vi "Test Panel.vi"() -> ()   [LabVIEW 2016]
uses:
  typedefs/Controlword--enum.ctl
  typedefs/Controlword--cluster.ctl
  typedefs/Statusword--cluster.ctl
  typedefs/Statusword--enum.ctl
  Libraries/Modbus-Master/MB_PDU/MB_PDU_Cluster.ctl
  IgusMotorDrive.lvclass
  Libraries/Modbus-Master/MB Master.lvlib
panel:
  out "Command":T1={"Function Code"=1, "Data"=[], "RTU_DataBytes"=0} {"Data" format="%.0x"}
  out "Response":T1={"Function Code"=1, "Data"=[], "RTU_DataBytes"=0} {"Data" format="%.0x"}
  in  "Stop Button":bool
  in  "Tab Control":T2(tab)
  in  "IP address":string="10.130.56.165"
  in  "port (502)":u16=502
  in  "Receive":bool
  in  "Send":bool
  in  "Controlword":T3=enum."Fault Reset"
  out "Controlword Out":T4
  out "Statusword out":T5
  out "Status":T6
  in  "Refresh Home Status":bool
  out "Homed Success":bool
  out "Homed":bool
  in  "Home":bool
  out "Actual Position":i32
  in  "Refresh Move Status":bool
  out "New Setpoint":bool
  in  "Move":bool
  in  "Setpoint Deceleration":u32
  in  "Setpoint Acceleration":u32=10000
  in  "Setpoint Velocity":u32=10000
  in  "Setpoint Position":i32=1000
  out "Target Reached":bool
  # "|    |    |    |    |    |    |    |    |    |    |    |    |    |    |\n|    |    |    |    |    |    |    |    |    |    |    +----+----+----+- Byte 19 ... 22: data field\n|    |    |    |    |    |    |    |    |    +----+- Byte 17, 18: SDO object bytes, = 1 ... 4\n|    |    |    |    |    |    |    +----+- Byte 15, 16: starting address = 0\n|    |    |    |    |    |    + Byte 14: sub index\n|    |    |    |    +----+- Byte 12, 13: object index\n|    |    |    +- Byte 11: Node ID = 0\n|    |    +------ Byte 10: protocol option fields, reserve, = 0\n|    +------ Byte  9: protocol option fields, 0 = read, 1 = write\n+----------- Byte  8 : MEI type, Modbus TCP = 13 (0Dh)"
  # "Set IP Address Run VI, if no error in connection, goto Initialisation"
  # "Status is polled continuously.\n\n\"Not ready to switch on\" and \"Switch On Disabled\" tell you that you should RTM and set Drive Profile to Modbus TCP before you set DI7/Enable.\n\nDepending upon Status select a suitable Controlword based on the transitions in the table below.\n\nOnce you have reached Operation Enabled, you may proceed to the Homing Mode tab."
  # "Click Home, stage should start homing\n\nClick Refresh to check status"
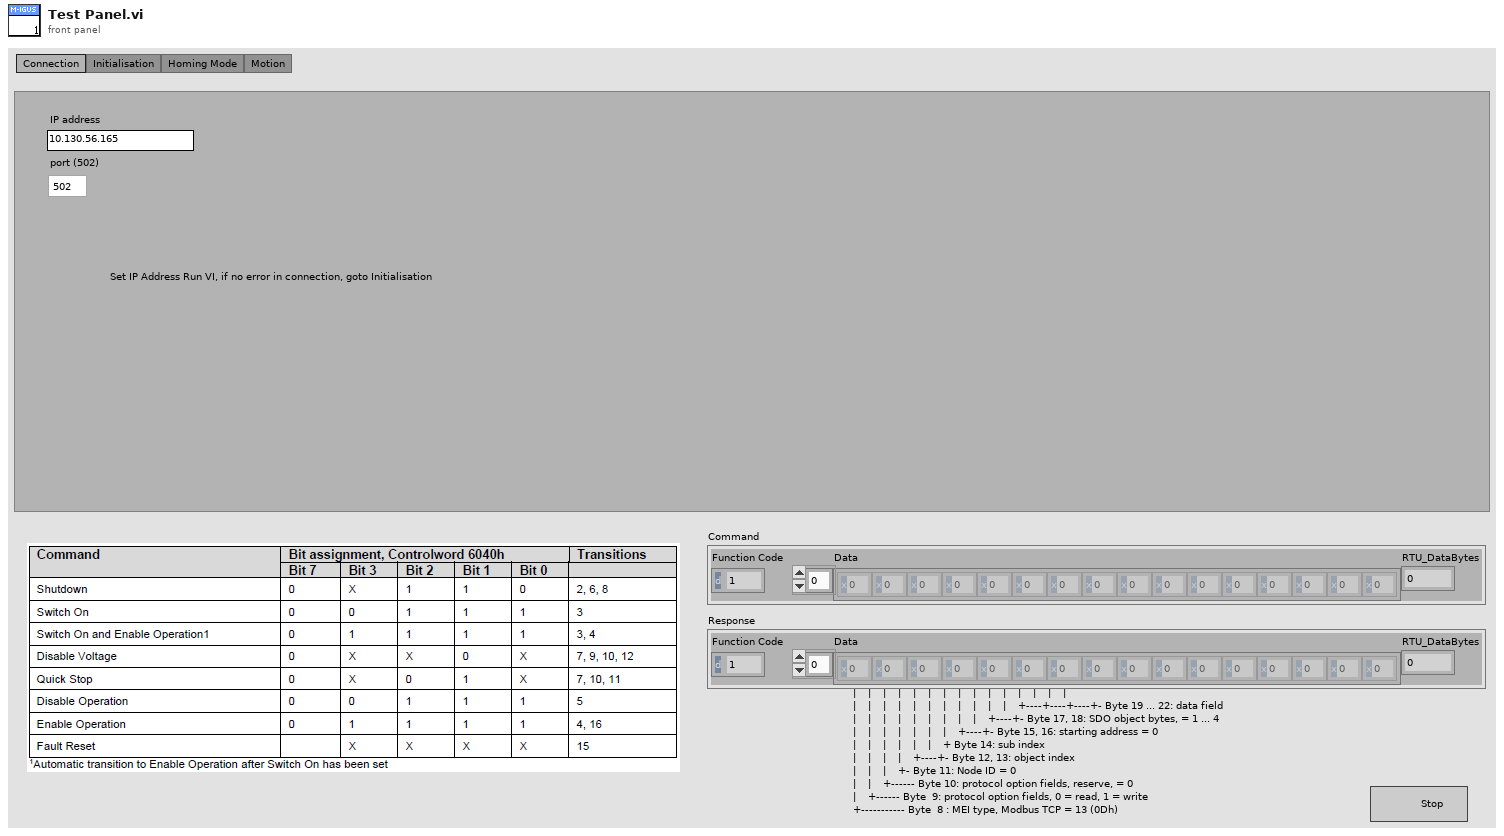
[diagram p1: front panel]
types:
  T1 = typedef "MB Master.lvlib/MB_PDU_Cluster.ctl" = cluster{"Function Code":u8, "Data":u8[], "RTU_DataBytes":i32}
  T2 = enum32{"Connection", "Initialisation", "Homing Mode", "Motion"}
  T3 = typedef "IgusMotorDrive.lvclass/Controlword--enum.ctl" = enum16{"Shutdown", "Switch On", "Switch On and Enable Operation", "Disable Voltage", "Quick Stop", "Disable Operation", "Enable Operation", "Fault Reset"}
  T4 = typedef "IgusMotorDrive.lvclass/Controlword--cluster.ctl" = cluster{"Switch On":bool, "Enable Voltage":bool, "Quick Stop":bool, "Enable Operation":bool, "4 MS (0: Homing Blocked/1: Homing Start) (0: No Start Signal/1: Start of Movement (0>1))":bool, "5 MS":bool, "6 MS(0:Absolute Positioning/1:Relative Positioning)":bool, "Fault Reset":bool, "Stop":bool, "9 MS":bool, "10 Reserved":bool, "11 Manufacturer Specific":bool, "12 Manufacturer Specific":bool, "13 Manufacturer Specific":bool, "14 Manufacturer Specific":bool, "15 Manufacturer Specific":bool}
  T5 = typedef "IgusMotorDrive.lvclass/Statusword--cluster.ctl" = cluster{"Ready to Switch On":bool, "Switched On":bool, "Operation Enabled":bool, "Fault":bool, "Voltage Enabled":bool, "Quick Stop":bool, "Switch On Disabled":bool, "Warning":bool, "8 Manufacturer Specific":bool, "Remote":bool, "Home Successful/Target Reached":bool, "Internal Limit Active":bool, "12 MS (0:Homing/1:Homed)":bool, "13 MS":bool, "14 Manufacturer Specific":bool, "15 Manufacturer Specific":bool}
  T6 = typedef "IgusMotorDrive.lvclass/Statusword--enum.ctl" = enum16{"Not Ready to Switch On", "Switch On Disabled", "Ready to Switch On", "Switched On", "Operation Enabled", "Quick Stop Active", "Fault Reaction Active", "Fault", "<Unknown>"}
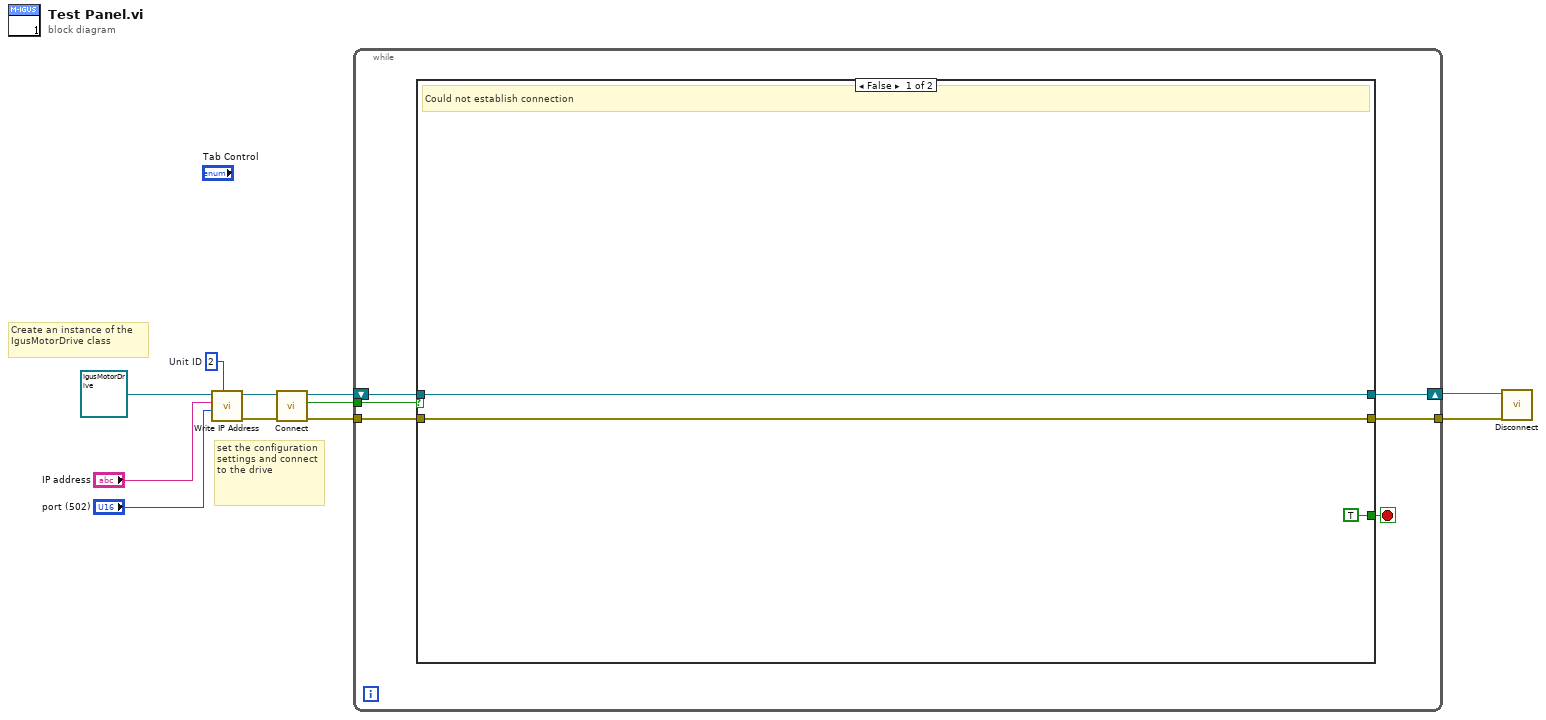
[diagram p0: block diagram]
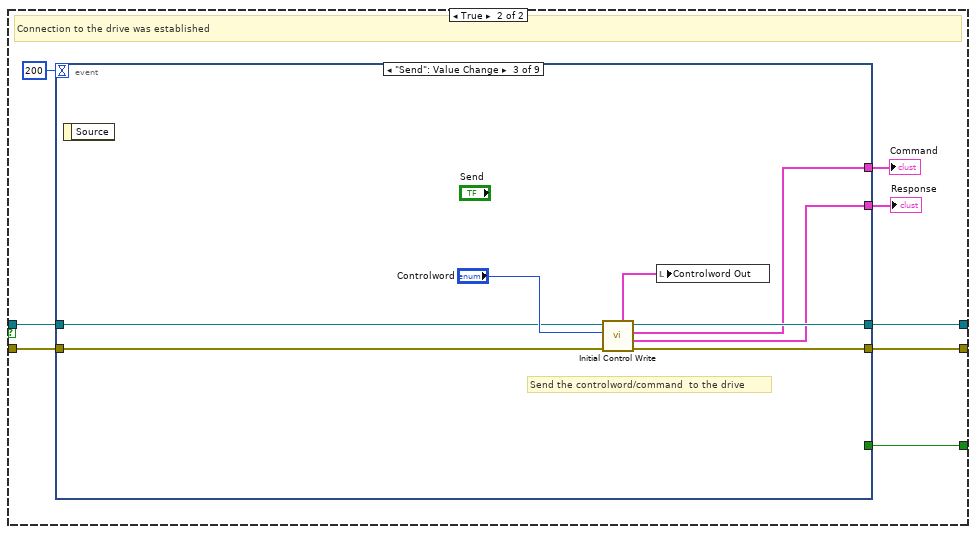
[diagram p2: hidden frame]
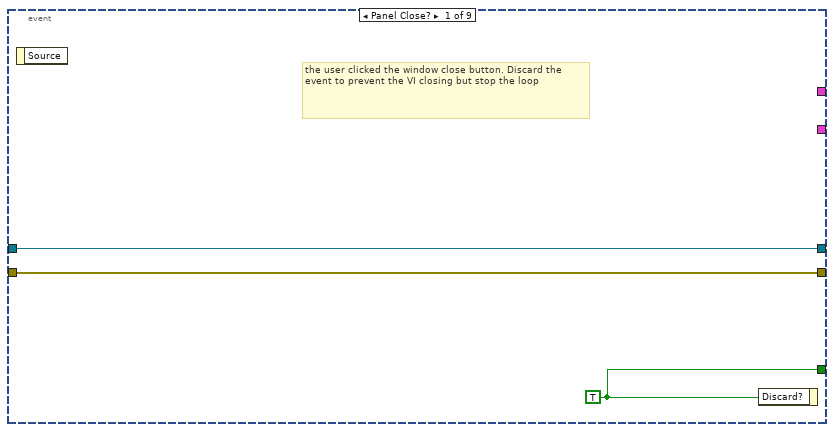
[diagram p3: hidden frame]
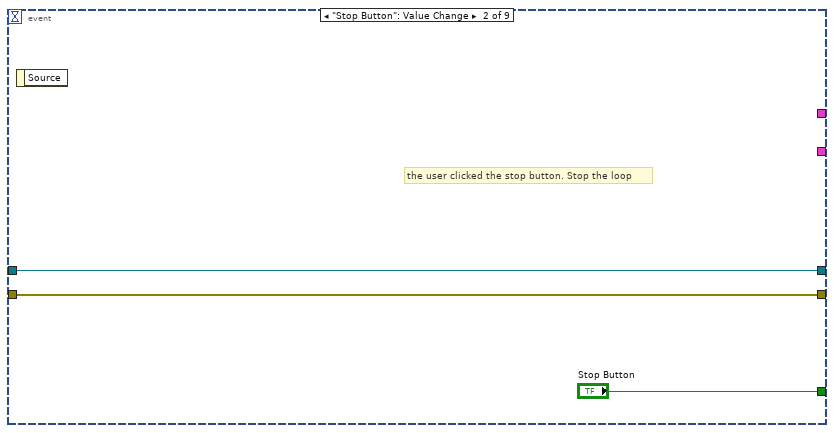
[diagram p4: hidden frame]
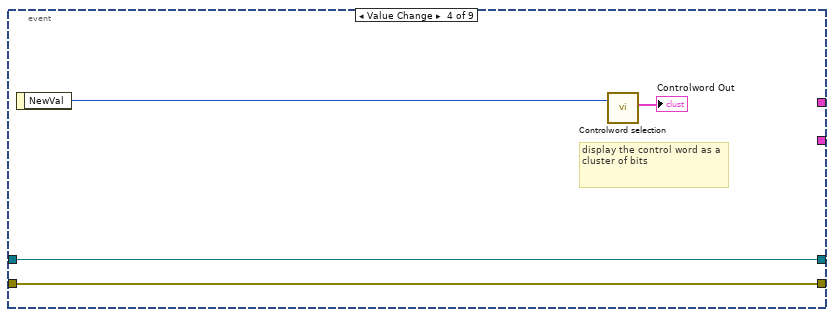
[diagram p5: hidden frame]
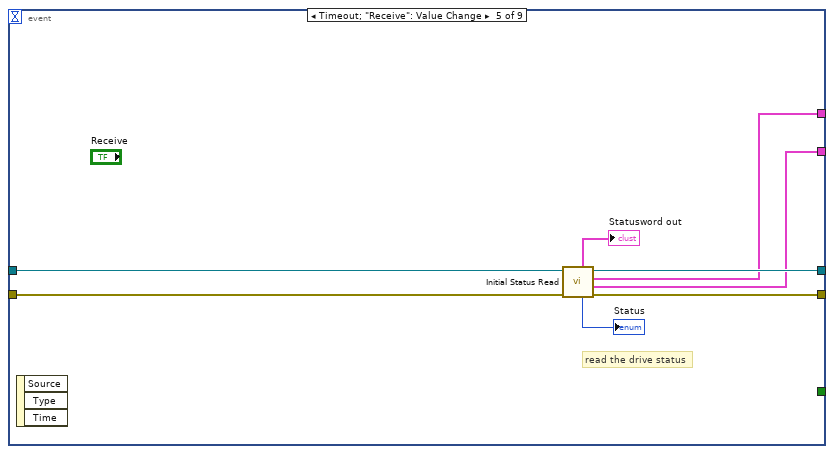
[diagram p6: hidden frame]
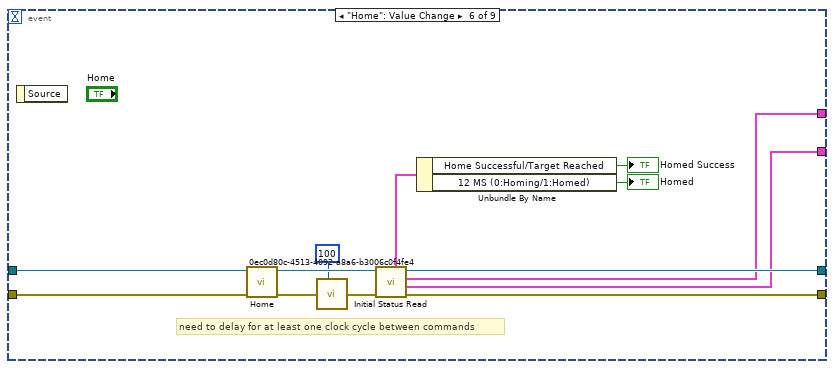
[diagram p7: hidden frame]
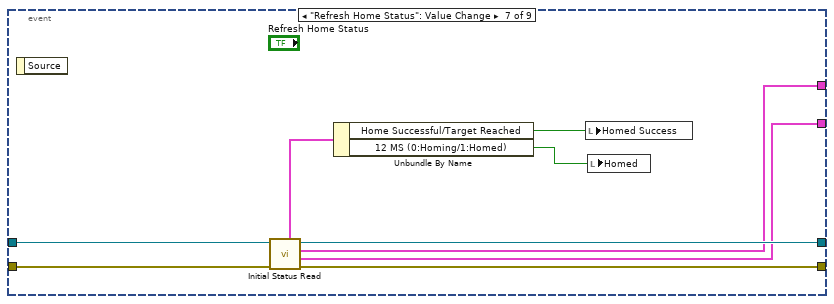
[diagram p8: hidden frame]
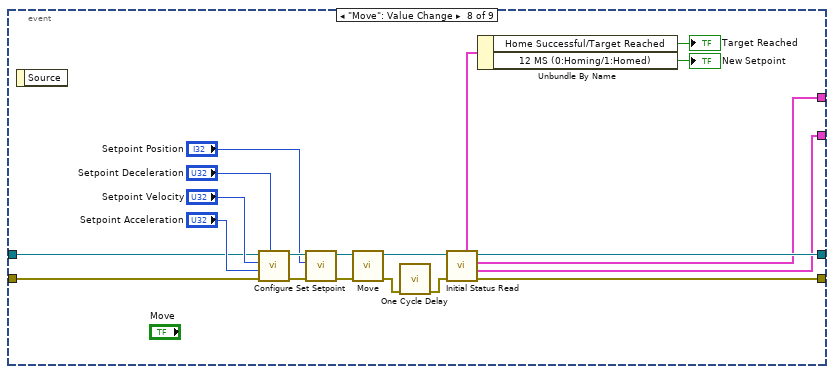
[diagram p9: hidden frame]
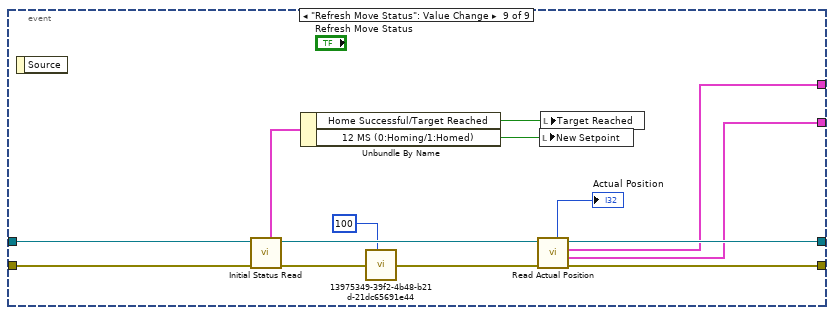
[diagram p10: hidden frame]
diagram:
  w6 = u8 2  # Unit ID
  # "set the configuration settings and connect to the drive"
  # "Create an instance of the IgusMotorDrive class"
  n1 = call-dynamic "Write IP Address.vi"("Unit ID"=w6, "Port"="port (502)", "IP Address"="IP address", "IgusMotorDrive in"=refnum<class "IgusMotorDrive.lvclass"> refnum) -> ("error out"=w7:errorcluster, "IgusMotorDrive out"=w8:refnum<class "IgusMotorDrive.lvclass">)  [unwired: 6 in]
  n2 = call-dynamic "Connect.vi"("error in (no error)"=w7, "IgusMotorDrive in"=w8) -> ("error out"=w4:errorcluster, "Is Connected"=w3:bool, "IgusMotorDrive out"=w2:refnum<class "IgusMotorDrive.lvclass">)  [unwired: 7 in]
  n3 = while {
    shift-right: [w13] -> w1
    shift-left: w2 -> [w16]
    tunnel: [w12] -> w11
    tunnel: w4 -> [w14]
    tunnel: w3 -> [w15]
    stop <- w17 stop-if-true
    n4 = case shown="False" w15 {
      tunnel: [TRUE ("Stop Button") w28] -> w17
      tunnel: w16 -> [w20 w27]
      tunnel: w14 -> [w19 w24]
      tunnel: [w20 w23] -> w13
      tunnel: [w19 w22] -> w12
      frame False {
        # "Could not establish connection"
      }
      frame True {
        # "Connection to the drive was established"
        n5 = event shown="[2] \"Send\": Value Change" {
          selector: _ -> [_ _ _ _ _ _ _ _ _]
          dyn-events: _ -> [_ _ _ _ _ _ _ _ _]
          timeout: 200 -> [_ _ _ _ _ _ _ _ _]
          tunnel: [w31 "Stop Button" _ _ _ _ _ _ _] -> w28
          tunnel: [w30 w33 w42 w44 w54 w65 w75 w90 w105] -> w23
          tunnel: w27 -> [w30 w33 w36 w44 w48 w57 w69 w78 w99]
          tunnel: [w29 w32 w40 w43 w53 w66 w76 w89 w107] -> w22
          tunnel: [_ _ w39 _ w52 w59 w71 w80 w103] -> w26
          tunnel: [_ _ w38 _ w51 w58 w70 w79 w102] -> w25
          tunnel: w24 -> [w29 w32 w35 w43 w47 w56 w68 w77 w98]
          event Panel Close? {
            w31 = TRUE
            # "the user clicked the window close button. Discard the event to prevent the VI closing but stop the loop"
            n6 = event-data() -> ()  [unwired: 1 in, 1 out]
            n7 = event-data("Discard?"=w31) -> ()  [unwired: 1 in, 1 out]
          }
          event "Stop Button": Value Change {
            # "the user clicked the stop button. Stop the loop"
            n8 = event-data() -> ()  [unwired: 1 in, 1 out]
          }
          event "Send": Value Change {
            # "Send the controlword/command  to the drive"
            n9 = event-data() -> ()  [unwired: 1 in, 1 out]
            n10 = call "Initial Control Write.vi"("error in (no error)"=w35, "Controlword"="Controlword", "IgusMotorDrive in"=w36) -> ("error out"=w40:errorcluster, "Response"=w38:T1, "Command"=w39:T1, "IgusMotorDrive out"=w42:refnum<class "IgusMotorDrive.lvclass">, "Controlword Out"=w37:T4)  [unwired: 4 in]
            n11 = local write "Controlword Out"(w37) -> ()
          }
          event Value Change {
            # "display the control word as a cluster of bits"
            n12 = event-data() -> ("NewVal"=w45:T3)  [unwired: 1 in]
            n13 = call "Controlword selection.vi"("Controlword"=w45) -> ("Controlword Out"=→"Controlword Out":T4)  [unwired: 7 in, 3 out]
          }
          event Timeout; "Receive": Value Change {
            # "read the drive status"
            n14 = event-data() -> ()  [unwired: 1 in, 3 out]
            n15 = call "Initial Status Read.vi"("error in (no error)"=w47, "IgusMotorDrive in"=w48) -> ("error out"=w53:errorcluster, "Response"=w51:T1, "Command"=w52:T1, "IgusMotorDrive out"=w54:refnum<class "IgusMotorDrive.lvclass">, "Statusword"=→"Status":T6, "Statusword out"=→"Statusword out":T5)  [unwired: 4 in]
          }
          event "Home": Value Change {
            # "need to delay for at least one clock cycle between commands"
            n16 = event-data() -> ()  [unwired: 1 in, 1 out]
            n17 = call-dynamic "Home.vi"("error in"=w56, "IgusMotorDrive in"=w57) -> ("error out"=w62:errorcluster, "IgusMotorDrive out"=w67:refnum<class "IgusMotorDrive.lvclass">)  [unwired: 8 in]
            n18 = call "0ec0d80c-4513-4092-a8a6-b3006c0f4fe4.vi"("value in"=w62, "milliseconds to wait"=u32 100) -> ("value out"=w61:errorcluster)  [unwired: 1 out]
            n19 = call "Initial Status Read.vi"("error in (no error)"=w61, "IgusMotorDrive in"=w67) -> ("error out"=w66:errorcluster, "Response"=w58:T1, "Command"=w59:T1, "IgusMotorDrive out"=w65:refnum<class "IgusMotorDrive.lvclass">, "Statusword out"=w60:T5)  [unwired: 4 in, 1 out]
            n20 = Unbundle By Name(w60) -> ("Home Successful/Target Reached"=→"Homed Success":bool, "12 MS (0:Homing/1:Homed)"=→"Homed":bool)
          }
          event "Refresh Home Status": Value Change {
            n21 = event-data() -> ()  [unwired: 1 in, 1 out]
            n22 = call "Initial Status Read.vi"("error in (no error)"=w68, "IgusMotorDrive in"=w69) -> ("error out"=w76:errorcluster, "Response"=w70:T1, "Command"=w71:T1, "IgusMotorDrive out"=w75:refnum<class "IgusMotorDrive.lvclass">, "Statusword out"=w72:T5)  [unwired: 4 in, 1 out]
            n23 = Unbundle By Name(w72) -> ("Home Successful/Target Reached"=w73:bool, "12 MS (0:Homing/1:Homed)"=w74:bool)
            n24 = local write "Homed Success"(w73) -> ()
            n25 = local write "Homed"(w74) -> ()
          }
          event "Move": Value Change {
            n26 = event-data() -> ()  [unwired: 1 in, 1 out]
            n27 = call-dynamic "Configure.vi"("Setpoint Deceleration"="Setpoint Deceleration", "error in (no error)"=w77, "Setpoint Acceleration"="Setpoint Acceleration", "Setpoint Velocity"="Setpoint Velocity", "IgusMotorDrive in"=w78) -> ("error out"=w95:errorcluster, "IgusMotorDrive out"=w96:refnum<class "IgusMotorDrive.lvclass">)  [unwired: 5 in]
            n28 = call-dynamic "Set Setpoint.vi"("error in (no error)"=w95, "Setpoint Position"="Setpoint Position", "IgusMotorDrive in"=w96) -> ("error out"=w93:errorcluster, "IgusMotorDrive out"=w94:refnum<class "IgusMotorDrive.lvclass">)  [unwired: 7 in]
            n29 = call-dynamic "Move.vi"("error in (no error)"=w93, "IgusMotorDrive in"=w94) -> ("error out"=w92:errorcluster, "IgusMotorDrive out"=w91:refnum<class "IgusMotorDrive.lvclass">)  [unwired: 8 in]
            n30 = call "One Cycle Delay.vi"("error in"=w92) -> ("error out"=w88:errorcluster)  [unwired: 10 in]
            n31 = call "Initial Status Read.vi"("error in (no error)"=w88, "IgusMotorDrive in"=w91) -> ("error out"=w89:errorcluster, "Response"=w79:T1, "Command"=w80:T1, "IgusMotorDrive out"=w90:refnum<class "IgusMotorDrive.lvclass">, "Statusword out"=w81:T5)  [unwired: 4 in, 1 out]
            n32 = Unbundle By Name(w81) -> ("Home Successful/Target Reached"=→"Target Reached":bool, "12 MS (0:Homing/1:Homed)"=→"New Setpoint":bool)
          }
          event "Refresh Move Status": Value Change {
            n33 = event-data() -> ()  [unwired: 1 in, 1 out]
            n34 = call "Initial Status Read.vi"("error in (no error)"=w98, "IgusMotorDrive in"=w99) -> ("error out"=w101:errorcluster, "IgusMotorDrive out"=w106:refnum<class "IgusMotorDrive.lvclass">, "Statusword out"=w108:T5)  [unwired: 4 in, 3 out]
            n35 = Unbundle By Name(w108) -> ("Home Successful/Target Reached"=w110:bool, "12 MS (0:Homing/1:Homed)"=w109:bool)
            n36 = call "13975349-39f2-4b48-b21d-21dc65691e44.vi"("value in"=w101, "milliseconds to wait"=u32 100) -> ("value out"=w100:errorcluster)  [unwired: 1 out]
            n37 = call "Read Actual Position.vi"("error in (no error)"=w100, "IgusMotorDrive in"=w106) -> ("error out"=w107:errorcluster, "Response"=w102:T1, "Command"=w103:T1, "IgusMotorDrive out"=w105:refnum<class "IgusMotorDrive.lvclass">, "Position"=→"Actual Position":i32)  [unwired: 5 in]
            n38 = local write "New Setpoint"(w109) -> ()
            n39 = local write "Target Reached"(w110) -> ()
          }
        }
        "Command" <- w26
        "Response" <- w25
      }
    }
  }
  n40 = call-dynamic "Disconnect.vi"("error in (no error)"=w11, "IgusMotorDrive in"=w1) -> ()  [unwired: 8 in, 2 out]
